vi "Index not Created for lvclass.vi"(8 "error in (no error)":errorcluster, 11 "Indexing Test Finder Test in":refnum<class "Indexing Test Finder Test.lvclass">) -> (0 "error out":errorcluster, 3 "Indexing Test Finder Test out":refnum<class "Indexing Test Finder Test.lvclass">)   [LabVIEW 2020, in "LUnit Tests.lvlib" / "Indexing Test Finder Test.lvclass"]
uses:
  Indexing Test Finder Test.lvclass
  Indexing Test Finder Test.lvclass/Indexing Test Finder Test.ctl
  source/Framework/Helper Classes/Test Finder/Test Finder.lvclass
  Test Finder/Finder Test.lvclass
  c59a45e6-8387-4d73-9fe8-839093b27eb6.vi
  Test Dummys/Test Test Case/Test Test Case.lvclass
  <vilib>/Astemes/LUnit/Test Case.lvclass
  C:/Git/astemes-lunit/source/Framework/Test Case/LUnit Test Case.lvclass
  C:/Git/astemes-lunit/tests/Test Dummys/Test Test Case/Test Test Case.lvclass
  C:/Git/astemes-lunit/tests/Test Finder/Finder Test.lvclass
  C:/Program Files (x86)/National Instruments/LabVIEW 2020/vi.lib/Astemes/LUnit/Test Case.lvclass
  C:/Git/astemes-lunit/tests/Indexing Test Finder Test/Indexing Test Finder Test.lvclass
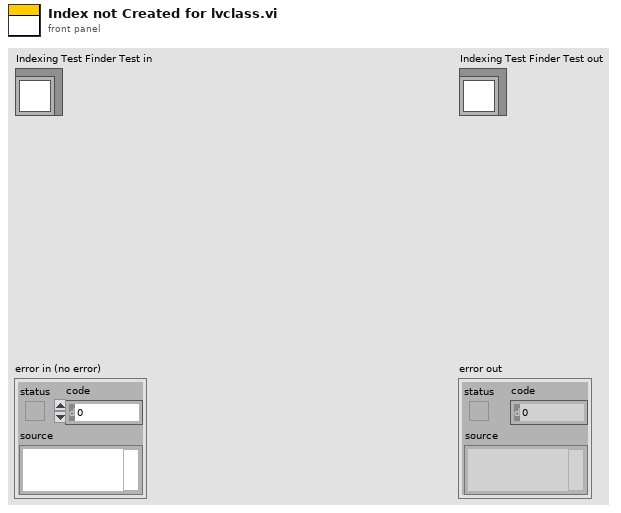
[diagram p1: front panel]
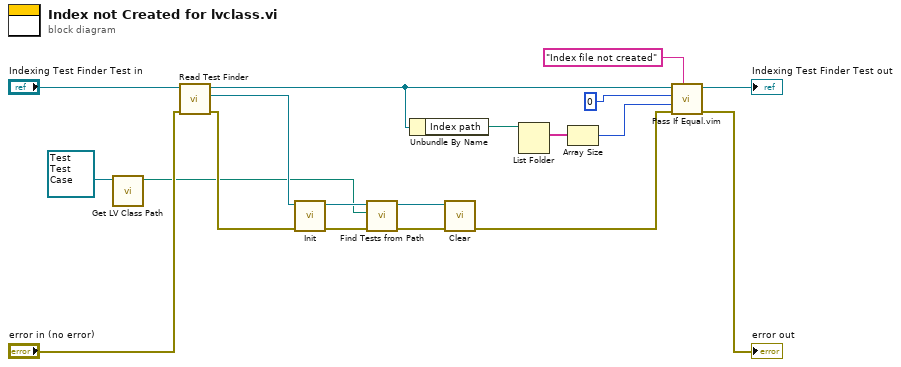
[diagram p0: block diagram]
diagram:
  n1 = call <vilib>:"Get LV Class Path.vi"("object"=refnum<class "Test Test Case.lvclass"> refnum ("Test Test Case.lvclass")) -> ("class path"=w1:path)  [unwired: 9 in, 1 out]
  n2 = call "Read Test Finder.vi"("error in (no error)"="error in (no error)", "Test Finder In"="Indexing Test Finder Test in") -> ("error out"=w13:errorcluster, "Test Finder.lvclass"=w14:refnum<class "Test Finder.lvclass">, "Test Finder Out"=w6:refnum<class "Indexing Test Finder Test.lvclass">)  [unwired: 7 in]
  n3 = call-dynamic "Init.vi"("error in (no error)"=w13, "Test Finder in"=w14) -> ("error out"=w17:errorcluster, "Test Finder out"=w18:refnum<class "Test Finder.lvclass">)  [unwired: 8 in]
  n4 = call-dynamic "Find Tests from Path.vi"("error in (no error)"=w17, "Project or Class Path"=w1, "Test Case Finder In"=w18) -> ("error out"=w15:errorcluster, "Test Case Finder Out"=w16:refnum<class "Test Finder.lvclass">)  [unwired: 7 in]
  n5 = Unbundle By Name(w6) -> ("Index path"=w10:path)
  n6 = call "Clear.vi"("error in (no error)"=w15, "Test Finder in"=w16) -> ("error out"=w11:errorcluster)  [unwired: 8 in, 1 out]
  n7 = List Folder(path=w10) -> (filenames=w9:string[])  [unwired: 3 in, 3 out]
  n8 = Array Size(array=w9) -> (size(s)=w5:i32)
  n9 = call "Pass If Equal.vim"("Description"="Index file not created", "error in (no error)"=w11, "Actual"=w5, "Expected"=0 ("size(s)"), "LUnit Test Case In"=w6) -> ("error out"=→"error out":errorcluster, "LUnit Test Case Out"=→"Indexing Test Finder Test out":refnum<class "Indexing Test Finder Test.lvclass">)  [unwired: 5 in]
